vi "tap_stim_rec_async.vi"(0 "Convert Power to Voltage B":bool, 2 "voltages/power B":dbl[](array[numeric]), 3 "SSH password":string, 4 "Transfer and Run Date Folder After Experiment":bool, 5 "SSH user name":string, 6 "Tags":string, 7 "Frames":i32, 8 "Convert Power to Voltage":bool, 9 "voltages/power A":dbl[](array[numeric]), 10 "parameters":string[](array[string]), 11 "parameters headers":string[](array[string])) -> ()   [LabVIEW 2014]
uses:
  <vilib>/vision/driver/IMAQdx.llb/IMAQdx Acquisition Mode.ctl
  <vilib>/userdefined/High Color/IMAQdx.ctl
  <vilib>/vision/driver/IMAQdx.llb/IMAQdx Buffer Number Mode.ctl
  <vilib>/Utility/file.llb/Write To Spreadsheet File (DBL).vi
  <vilib>/Utility/file.llb/Write To Spreadsheet File (string).vi
  <vilib>/Utility/file.llb/Read From Spreadsheet File (string).vi
  <vilib>/vision/driver/NI_Vision_Acquisition_Software.lvlib
panel:
  out "Waveform Graph":dbl[](graph)
  out "Current Voltage B":dbl
  out "Current Voltage A":dbl
  out "Saved Buffer Number":u32
  out "ProcessFrameRate":dbl
  out "# elements in queue":i32
  out "CameraFrameRate":dbl
  out "Camera Buffer Number":u32
  out "Image":T1(plugin-control)
  out "JPEG Quality":dbl
  out "Error":string
  out "Save Directory":path
  in  "stop":bool
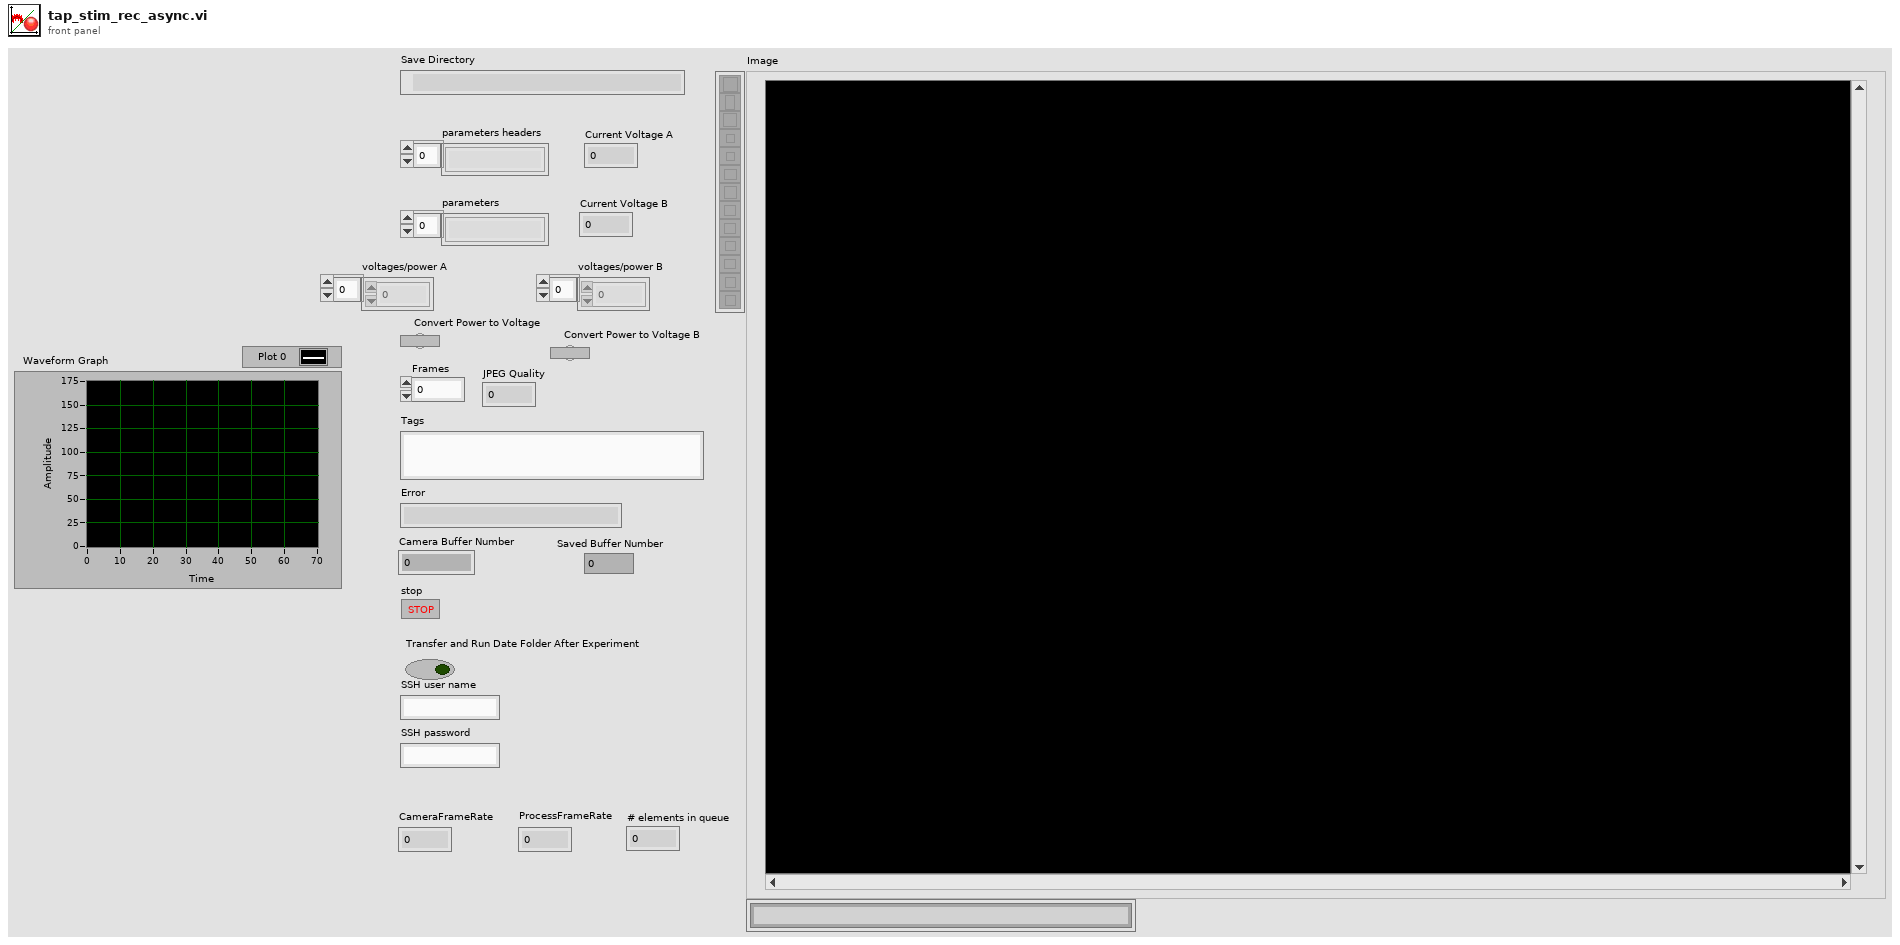
[diagram p1: front panel]
types:
  T1 = typedef "IMAQ Image.ctl" = refnum<image>
  T2 = typedef "IMAQdx.ctl" = refnum<k21>
  T3 = typedef "NI_Vision_Acquisition_Software.lvlib/IMAQdx Buffer Number Mode.ctl" = enum32{"Next", "Last", "Buffer Number"}
  T4 = typedef "Image Type" = u32
  T5 = typedef "NI_Vision_Acquisition_Software.lvlib/IMAQdx Acquisition Mode.ctl" = enum32{"One Shot", "Continuous"}
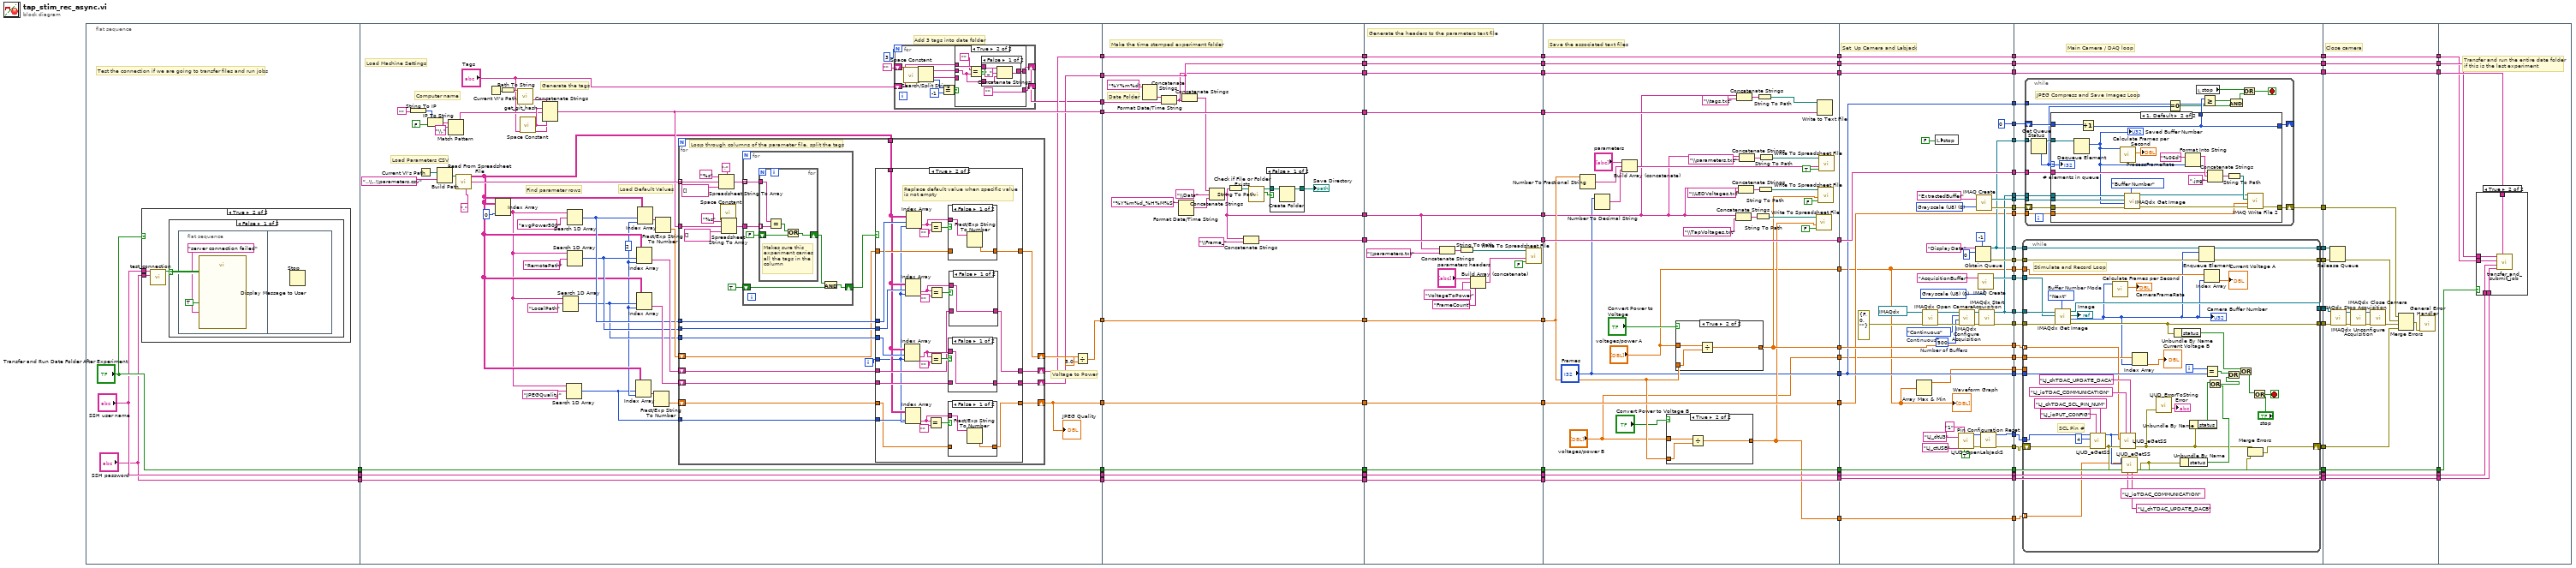
[diagram p0: block diagram]
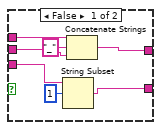
[diagram p4: hidden frame]
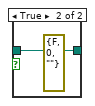
[diagram p11: hidden frame]
diagram:
  n1 = flat-sequence {
    tunnel: ["Transfer and Run Date Folder After Experiment"] -> w55
    tunnel: ["SSH user name"] -> w54
    tunnel: ["SSH password"] -> w53
    tunnel: [w139] -> w85
    tunnel: [w122] -> w84
    tunnel: [w113] -> w75
    tunnel: [w114] -> w74
    tunnel: w55 -> [w131]
    tunnel: w54 -> [w130]
    tunnel: w53 -> [w129]
    tunnel: [w131] -> w46
    tunnel: [w130] -> w39
    tunnel: [w129] -> w38
    tunnel: [w110] -> w31
    tunnel: [w101] -> w30
    tunnel: [w275] -> w69
    tunnel: [w274] -> w67
    tunnel: [w273] -> w65
    tunnel: [w272] -> w63
    tunnel: [w254] -> w61
    tunnel: [w256] -> w59
    tunnel: [w271] -> w57
    tunnel: w74 -> [w271]
    tunnel: w75 -> [w256]
    tunnel: w84 -> [w272]
    tunnel: w85 -> [w273]
    tunnel: [w263] -> w47
    tunnel: w46 -> [w263]
    tunnel: [w262] -> w40
    tunnel: w39 -> [w262]
    tunnel: w38 -> [w261]
    tunnel: [w261] -> w37
    tunnel: w31 -> [w257]
    tunnel: w30 -> [w253]
    tunnel: [w253] -> w27
    tunnel: w69 -> [w297]
    tunnel: [w297] -> w68
    tunnel: w67 -> [w283]
    tunnel: [w283] -> w66
    tunnel: w65 -> [w296]
    tunnel: [w296] -> w64
    tunnel: w63 -> [w295]
    tunnel: [w295] -> w62
    tunnel: w61 -> [w294]
    tunnel: [w294] -> w60
    tunnel: w59 -> [w293]
    tunnel: [w293] -> w58
    tunnel: w57 -> [w292]
    tunnel: [w292] -> w56
    tunnel: [w282] -> w48
    tunnel: w47 -> [w282]
    tunnel: [w281] -> w41
    tunnel: w40 -> [w281]
    tunnel: w37 -> [w280]
    tunnel: [w280] -> w36
    tunnel: [w279] -> w28
    tunnel: w27 -> [w279]
    tunnel: w68 -> [w332]
    tunnel: [w332] -> w90
    tunnel: [w302] -> w88
    tunnel: ["Frames"] -> w87
    tunnel: w66 -> [w303]
    tunnel: w64 -> [w309]
    tunnel: w62 -> [w312]
    tunnel: w60 -> [w321]
    tunnel: [w321] -> w80
    tunnel: [w320] -> w76
    tunnel: w58 -> [w320]
    tunnel: [w319] -> w70
    tunnel: w56 -> [w319]
    tunnel: [w315] -> w49
    tunnel: w48 -> [w315]
    tunnel: [w314] -> w42
    tunnel: w41 -> [w314]
    tunnel: w36 -> [w313]
    tunnel: [w313] -> w35
    tunnel: [w311] -> w29
    tunnel: w28 -> [w311]
    tunnel: [w301] -> w6
    tunnel: ["voltages/power A"] -> w5
    tunnel: ["voltages/power B"] -> w3
    tunnel: w90 -> [w352]
    tunnel: [w382] -> w92
    tunnel: [w381] -> w91
    tunnel: [w385] -> w89
    tunnel: w88 -> [w385]
    tunnel: w87 -> [w351]
    tunnel: [w351] -> w86
    tunnel: [w379] -> w81
    tunnel: w80 -> [w379]
    tunnel: [w378] -> w77
    tunnel: w76 -> [w378]
    tunnel: [w377] -> w71
    tunnel: w70 -> [w377]
    tunnel: [w376] -> w50
    tunnel: w49 -> [w376]
    tunnel: [w375] -> w43
    tunnel: w42 -> [w375]
    tunnel: w35 -> [w374]
    tunnel: [w374] -> w34
    tunnel: w29 -> [w349]
    tunnel: [w358] -> w26
    tunnel: [w353] -> w25
    tunnel: [w357] -> w24
    tunnel: [w356] -> w23
    tunnel: [w350] -> w22
    tunnel: [w355] -> w19
    tunnel: [w354] -> w18
    tunnel: [w353] -> w17
    tunnel: [w352] -> w16
    tunnel: [w351] -> w15
    tunnel: [w350] -> w14
    tunnel: [w349] -> w13
    tunnel: [0] -> w9
    tunnel: [w346] -> w7
    tunnel: w6 -> [w346]
    tunnel: w5 -> [w344]
    tunnel: [w344] -> w4
    tunnel: w3 -> [w345]
    tunnel: [w345] -> w2
    tunnel: [w343] -> w1
    tunnel: w92 -> [w406]
    tunnel: w91 -> [w398]
    tunnel: w89 -> [w404]
    tunnel: w86 -> [w405]
    tunnel: [w421] -> w82
    tunnel: w81 -> [w421]
    tunnel: [w420] -> w78
    tunnel: w77 -> [w420]
    tunnel: [w419] -> w72
    tunnel: w71 -> [w419]
    tunnel: [w418] -> w51
    tunnel: w50 -> [w418]
    tunnel: [w417] -> w44
    tunnel: w43 -> [w417]
    tunnel: w34 -> [w416]
    tunnel: [w416] -> w33
    tunnel: w26 -> [w399]
    tunnel: w25 -> [w400]
    tunnel: w24 -> [w401]
    tunnel: w23 -> [w402]
    tunnel: w22 -> [w403]
    tunnel: [w394] -> w21
    tunnel: [w393] -> w20
    tunnel: w19 -> [w415]
    tunnel: w18 -> [w414]
    tunnel: w17 -> [w413]
    tunnel: w16 -> [w412]
    tunnel: w15 -> [w411]
    tunnel: w14 -> [w410]
    tunnel: w13 -> [w409]
    tunnel: [w392] -> w12
    tunnel: [w395] -> w11
    tunnel: [w408] -> w10
    tunnel: w9 -> [w407]
    tunnel: [w396] -> w8
    tunnel: w7 -> [w397]
    tunnel: w4 -> [w391]
    tunnel: w2 -> [w390]
    tunnel: w1 -> [w389]
    tunnel: [w524] -> w83
    tunnel: w82 -> [w524]
    tunnel: [w523] -> w79
    tunnel: w78 -> [w523]
    tunnel: [w522] -> w73
    tunnel: w72 -> [w522]
    tunnel: [w521] -> w52
    tunnel: w51 -> [w521]
    tunnel: [w520] -> w45
    tunnel: w44 -> [w520]
    tunnel: w33 -> [w519]
    tunnel: [w519] -> w32
    tunnel: w21 -> [w514]
    tunnel: w20 -> [w513]
    tunnel: w12 -> [w508]
    tunnel: w11 -> [w511]
    tunnel: w10 -> [w510]
    tunnel: w8 -> [w509]
    tunnel: w83 -> [w530]
    tunnel: w79 -> [w529]
    tunnel: w73 -> [w528]
    tunnel: w52 -> [w527]
    tunnel: w45 -> [w526]
    tunnel: w32 -> [w525]
    frame #0 {
      # "Test the connection if we are going to transfer files and run jobs"
      n2 = case shown="True" "Transfer and Run Date Folder After Experiment" {
        tunnel: "SSH password" -> [_ w98]
        tunnel: "SSH user name" -> [_ w96]
        frame False {
        }
        frame True {
          n3 = call "test_connection.vi"("Username"=w96, "Password"=w98) -> ("Connection Successful"=w97:bool)  [unwired: 7 in]
          n4 = case shown="False" w97 {
            frame False {
              n5 = flat-sequence {
                frame #0 {
                  n6 = call "Display Message to User"("Enable"=TRUE, "Message"="server connection failed") -> ()  [unwired: 8 in, 2 out]
                }
                frame #1 {
                  n7 = Stop() -> ()  [unwired: 1 in]
                }
              }
            }
            frame True {
            }
          }
        }
      }
    }
    frame #1 {
      w104 = 2
      # "Add 3 tags into date folder"
      # "Generate the tags"
      # "Find parameter rows"
      # "Load Default Values"
      # "Voltage to Power"
      # "Load Parameters CSV"
      # "Computer name"
      # "Load Machine Settings"
      n8 = String To IP(1:"") -> (0:w147:u32)
      n9 = Current VI's Path() -> (path=w142:path)
      n10 = IP To String(1:FALSE, 2:w147) -> (0:w144:string)
      n11 = Build Path(base path=w142, name or relative path="..\\..\\parameters.csv") -> (appended path=w133:path)
      n12 = Match Pattern(string=w144, regular expression="\\.") -> (before substring=w124:string)  [unwired: 1 in, 3 out]
      n13 = call-poly <vilib>:"Read From Spreadsheet File.vi"("delimiter (\\t)"=",", "file path (dialog if empty)"=w133) -> ("first row"=w123:string[], "all rows"=w106:string[][])  [unwired: 5 in, 3 out]
      n14 = Current VI's Path() -> (path=w126:path)
      n15 = Index Array(array=w106, index (col)=0) -> (element=w105:string[])  [unwired: 1 in]
      n16 = Path To String(path=w126) -> (string=w125:string)
      n17 = call "get_git_hash.vi"("VI folder"=w125) -> ("github hash"=w128:string)  [unwired: 10 in]
      n18 = call <vilib>:"Space Constant.vi"() -> ("String"=w127:string)
      n19 = Concatenate Strings(w128, w127, w124, w127, "Tags") -> (w122:string)
      n20 = Search 1D Array(1D array=w105, element="LocalPath") -> (index of element=w116:i32)  [unwired: 1 in]
      n21 = Search 1D Array(1D array=w105, element="JPEGQuality") -> (index of element=w102:i32)  [unwired: 1 in]
      n22 = Search 1D Array(1D array=w105, element="RemotePath") -> (index of element=w117:i32)  [unwired: 1 in]
      n23 = Search 1D Array(1D array=w105, element="avgPower500") -> (index of element=w118:i32)  [unwired: 1 in]
      n24 = Index Array(array=w106, index (row)=w102, index (col)=w104) -> (element=w107:string)
      n25 = Index Array(array=w106, index (row)=w117, index (col)=w104) -> (element=w120:string)
      n26 = Index Array(array=w106, index (row)=w116, index (col)=w104) -> (element=w119:string)
      n27 = Index Array(array=w106, index (row)=w118, index (col)=w104) -> (element=w135:string)
      n28 = Fract/Exp String To Number(string=w107) -> (number=w103:dbl)  [unwired: 3 in, 1 out]
      n29 = Fract/Exp String To Number(string=w135) -> (number=w121:dbl)  [unwired: 3 in, 1 out]
      n30 = for {
        tunnel: w123 -> [w201] mode=indexing
        tunnel: w122 -> [w193]
        tunnel: w118 -> [w188]
        tunnel: w117 -> [w187]
        tunnel: w116 -> [w186]
        tunnel: w106 -> [w191]
        shift-right: [w183] -> w115
        shift-left: w121 -> [w184]
        shift-right: [w180] -> w114
        shift-left: w120 -> [w181]
        shift-right: [w179] -> w113
        shift-left: w119 -> [w182]
        shift-right: [w176] -> w101
        shift-left: w103 -> [w178]
        tunnel: w102 -> [w177]
        i -> [w185]
        # "Loop through columns of the parameter file, split the tags"
        n31 = Spreadsheet String To Array(delimiter (Tab)=";", format string="%s", spreadsheet string=w201, array type (2D Dbl)=string[] []) -> (array=w197:string[])
        n32 = call <vilib>:"Space Constant.vi"() -> ("String"=w195:string)
        n33 = Spreadsheet String To Array(delimiter (Tab)=w195, format string="%s", spreadsheet string=w193, array type (2D Dbl)=string[] []) -> (array=w192:string[])
        n34 = for {
          tunnel: w197 -> [w247] mode=indexing
          tunnel: w192 -> [w246]
          shift-right: [w244] -> w189
          shift-left: TRUE -> [w242]
          n35 = for {
            tunnel: w247 -> [w252]
            tunnel: w246 -> [w251] mode=indexing
            shift-right: [w248] -> w243
            shift-left: FALSE -> [w249]
            # "Makes sure this\nexperiment carries\nall the tags in the\ncolumn"
            n36 = Equal?(x=w252, y=w251) -> (x = y?=w250:bool)
            n37 = Or(x=w250, y=w249) -> (x .or. y?=w248:bool)
          }
          n38 = And(x=w243, y=w242) -> (x .and. y?=w244:bool)
        }
        n39 = case shown="True" w189 {
          tunnel: w184 -> [w205 w226]
          tunnel: [w205 w225] -> w183
          tunnel: w188 -> [_ w231]
          tunnel: w187 -> [_ w230]
          tunnel: w186 -> [_ w229]
          tunnel: w185 -> [_ w208]
          tunnel: w191 -> [_ w209]
          tunnel: [w204 w215] -> w180
          tunnel: [w203 w217] -> w179
          tunnel: w182 -> [w203 w216]
          tunnel: w181 -> [w204 w214]
          tunnel: w178 -> [w202 w206]
          tunnel: w177 -> [_ w207]
          tunnel: [w202 w210] -> w176
          frame False {
          }
          frame True {
            # "Replace default value when specific value\nis not empty"
            n40 = Index Array(array=w209, index (row)=w229, index (col)=w208) -> (element=w218:string)
            n41 = Index Array(array=w209, index (row)=w230, index (col)=w208) -> (element=w221:string)
            n42 = Index Array(array=w209, index (row)=w207, index (col)=w208) -> (element=w211:string)
            n43 = Index Array(array=w209, index (row)=w231, index (col)=w208) -> (element=w224:string)
            n44 = Equal?(x=w211, y="") -> (x = y?=w212:bool)
            n45 = Equal?(x=w224, y="") -> (x = y?=w227:bool)
            n46 = Equal?(x=w218, y="") -> (x = y?=w219:bool)
            n47 = Equal?(x=w221, y="") -> (x = y?=w222:bool)
            n48 = case shown="False" w212 {
              tunnel: w206 -> [_ w234]
              tunnel: [w233 w234] -> w210
              tunnel: w211 -> [w232 _]
              frame False {
                n49 = Fract/Exp String To Number(string=w232) -> (number=w233:dbl)  [unwired: 3 in, 1 out]
              }
              frame True {
              }
            }
            n50 = case shown="False" w227 {
              tunnel: w226 -> [_ w241]
              tunnel: [w240 w241] -> w225
              tunnel: w224 -> [w239 _]
              frame False {
                n51 = Fract/Exp String To Number(string=w239) -> (number=w240:dbl)  [unwired: 3 in, 1 out]
              }
              frame True {
              }
            }
            n52 = case shown="False" w219 {
              tunnel: w218 -> [w235 _]
              tunnel: [w235 w236] -> w217
              tunnel: w216 -> [_ w236]
              frame False {
              }
              frame True {
              }
            }
            n53 = case shown="False" w222 {
              tunnel: w221 -> [w237 _]
              tunnel: [w237 w238] -> w215
              tunnel: w214 -> [_ w238]
              frame False {
              }
              frame True {
              }
            }
          }
        }
      }
      "JPEG Quality" <- w101
      n54 = for {
        N: 3 -> [_]
        shift-right: [w148] -> _
        shift-left: "Tags" -> [w157]
        shift-right: [w150] -> w110
        shift-left: "" -> [w155]
        n55 = call <vilib>:"Space Constant.vi"() -> ("String"=w156:string)
        n56 = Search/Split String(string=w157, search string/char (-)=w156) -> (substring before match=w154:string, match + rest of string=w153:string, offset of match=w152:i32)  [unwired: 1 in]
        n57 = Equal?(x=w152, y=-1) -> (x = y?=w149:bool)
        n58 = case shown="True" w149 {
          tunnel: w155 -> [w158 w168]
          tunnel: w154 -> [w159 w165]
          tunnel: w153 -> [w160 _]
          tunnel: [w162 ""] -> w148
          tunnel: [w161 w167] -> w150
          frame False {
            n59 = String Subset(string=w160, offset (0)=1) -> (substring=w162:string)  [unwired: 1 in]
            n60 = Concatenate Strings(w158, "_", w159) -> (w161:string)
          }
          frame True {
            n61 = Equal?(x="", y=w165) -> (x = y?=w169:bool)
            n62 = case shown="False" w169 {
              tunnel: w168 -> [w172 w175]
              tunnel: [w173 w175] -> w167
              tunnel: w165 -> [w171 _]
              frame False {
                n63 = Concatenate Strings(w172, "_", w171) -> (w173:string)
              }
              frame True {
              }
            }
          }
        }
      }
      n64 = Divide(x=w115, y=5.0) -> (x/y=w139:dbl)
    }
    frame #2 {
      # "Make the time stamped experiment folder"
      # "Date Folder"
      n65 = Format Date/Time String(time format string (%c)="%Y%m%d") -> (date/time string=w258:string)  [unwired: 2 in]
      n66 = Concatenate Strings(w258, w257) -> (w254:string)
      n67 = Format Date/Time String(time format string (%c)="%Y%m%d_%H%M%S") -> (date/time string=w260:string)  [unwired: 2 in]
      n68 = Concatenate Strings(w256, w254) -> (w255:string)
      n69 = Concatenate Strings(w255, "\\Data", w260) -> (w274:string)
      n70 = String To Path(string=w274) -> (path=w266:path)
      n71 = Concatenate Strings(w274, "\\Frame_") -> (w275:string)
      n72 = call <vilib>:"Check if File or Folder Exists.vi"("path"=w266) -> ("file or folder exists?"=w269:bool, "dup path"=w268:path)  [unwired: 8 in, 1 out]
      n73 = case shown="False" w269 {
        tunnel: [w276 w278] -> w265
        tunnel: w268 -> [w277 w278]
        frame False {
          n74 = Create Folder(path (use dialog)=w277) -> (created path=w276:path)  [unwired: 2 in, 2 out]
        }
        frame True {
          (unwired) errorcluster {"status"=FALSE, "code"=0, "source"=""} ("error out")
        }
      }
      "Save Directory" <- w265
    }
    frame #3 {
      # "Generate the headers to the parameters text file"
      n75 = Concatenate Strings(w283, "\\parameters.txt") -> (w291:string)
      n76 = String To Path(string=w291) -> (path=w290:path)
      n77 = Build Array (concatenate)("parameters headers", "VoltageToPower", "FrameCount") -> (w287:string[])
      n78 = call-poly <vilib>:"Write To Spreadsheet File.vi"("append to file? (new file:F)"=FALSE, "1D data"=w287, "file path (dialog if empty)"=w290) -> ()  [unwired: 5 in, 1 out]
    }
    frame #4 {
      # "Save the associated text files"
      n79 = Number To Fractional String(number=w309) -> (F-format string=w316:string)  [unwired: 3 in]
      n80 = Number To Decimal String(number="Frames") -> (decimal integer string=w317:string)  [unwired: 1 in]
      n81 = Build Array (concatenate)("parameters", w316, w317) -> (w325:string[])
      n82 = case shown="True" "Convert Power to Voltage B" {
        tunnel: "voltages/power B" -> [w335 w338]
        tunnel: [w335 w336] -> w301
        tunnel: w309 -> [_ w337]
        frame False {
        }
        frame True {
          n83 = Divide(x=w338, y=w337) -> (x/y=w336:dbl[])
        }
      }
      n84 = case shown="True" "Convert Power to Voltage" {
        tunnel: "voltages/power A" -> [w339 w342]
        tunnel: [w339 w340] -> w302
        tunnel: w309 -> [_ w341]
        frame False {
        }
        frame True {
          n85 = Divide(x=w342, y=w341) -> (x/y=w340:dbl[])
        }
      }
      n86 = Concatenate Strings(w303, "\\TapVoltages.txt") -> (w307:string)
      n87 = Concatenate Strings(w303, "\\tags.txt") -> (w323:string)
      n88 = Concatenate Strings(w303, "\\LEDVoltages.txt") -> (w334:string)
      n89 = Concatenate Strings(w303, "\\parameters.txt") -> (w329:string)
      n90 = String To Path(string=w307) -> (path=w306:path)
      n91 = String To Path(string=w323) -> (path=w322:path)
      n92 = String To Path(string=w334) -> (path=w333:path)
      n93 = String To Path(string=w329) -> (path=w328:path)
      n94 = call-poly <vilib>:"Write To Spreadsheet File.vi"("append to file? (new file:F)"=FALSE, "1D data"=w301, "file path (dialog if empty)"=w306) -> ()  [unwired: 5 in, 1 out]
      n95 = Write to Text File(file (use dialog)=w322, text=w312) -> ()  [unwired: 2 in, 3 out]
      n96 = call-poly <vilib>:"Write To Spreadsheet File.vi"("append to file? (new file:F)"=FALSE, "1D data"=w302, "file path (dialog if empty)"=w333) -> ()  [unwired: 5 in, 1 out]
      n97 = call-poly <vilib>:"Write To Spreadsheet File.vi"("append to file? (new file:F)"=TRUE, "1D data"=w325, "file path (dialog if empty)"=w328) -> ()  [unwired: 5 in, 1 out]
    }
    frame #5 {
      w361 = T4 0 items=["Grayscale (U8)", "Grayscale (I16)", "Grayscale (SGL)", "Complex (CSG)", "RGB (U32)", "HSL (U32)", "RGB (U64)"] ("Image Type")
      w370 = T4 0 items=["Grayscale (U8)", "Grayscale (I16)", "Grayscale (SGL)", "Complex (CSG)", "RGB (U32)", "HSL (U32)", "RGB (U64)"] ("Image Type")
      w371 = u32 500  # Number of Buffers
      w367 = IMAQdx_Acquisition_Mode."Continuous"  # Continuous?
      # "Set  Up Camera and Labjack"
      n98 = Array Max & Min(array=w344) -> (max value=w343:dbl)  [unwired: 3 out]
      n99 = call <vilib>:"IMAQdx Open Camera.vi"("error in"=errorcluster {"status"=FALSE, "code"=0, "source"=""}, "Session In"=T2 "cam0") -> ("error out"=w372:errorcluster, "Session Out"=w373:T2)  [unwired: 8 in]
      n100 = local write "stop"(FALSE) -> ()
      n101 = call "LJUD_OpenLabJackS.vi"("FirstFound"=TRUE, "Address"="1" ("DeviceType"), "ConnectionType"="LJ_ctUSB", "DeviceType"="LJ_dtU3") -> ("error out"=w380:errorcluster, "Handle"=w383:i32)  [unwired: 5 in, 1 out]
      n102 = call <vilib>:"IMAQdx Configure Acquisition.vi"("error in"=w372, "Number of Buffers"=w371, "Continuous?"=w367, "Session In"=w373) -> ("error out"=w368:errorcluster, "Session Out"=w366:T2)  [unwired: 6 in]
      n103 = Obtain Queue(max queue size (-1, unlimited)=-1, name (unnamed)="DisplayData", element data type=u32 0) -> (queue out=w350:refnum<queue>, error out=w356:errorcluster)  [unwired: 2 in, 1 out]
      n104 = call "IMAQ Create"("Image Name"="ExtractedBuffer", "Image Type"=w361) -> ("New Image"=w354:T1, "error out"=w355:errorcluster)  [unwired: 3 in]
      n105 = call "IMAQ Create"("Image Name"="AcquisitionBuffer", "Image Type"=w370) -> ("New Image"=w357:T1)  [unwired: 3 in, 1 out]
      n106 = call <vilib>:"IMAQdx Start Acquisition.vi"("error in"=w368, "Session In"=w366) -> ("error out"=w358:errorcluster, "Session Out"=w353:T2)  [unwired: 8 in]
      n107 = call "Pin Configuration Reset.vi"("error in"=w380, "Handle In"=w383) -> ("error out"=w381:errorcluster, "Handle Out"=w382:i32)  [unwired: 8 in]
      "Waveform Graph" <- w344
    }
    frame #6 {
      # "Main Camera / DAQ loop"
      n108 = while {
        shift-right: [w427] -> w392
        shift-left: w398 -> [w455]
        tunnel: w404 -> [w454] mode=indexing
        tunnel: w405 -> [w461]
        tunnel: w399 -> [w450]
        tunnel: w400 -> [w449]
        tunnel: w401 -> [w448]
        tunnel: w402 -> [w447]
        tunnel: w403 -> [w446]
        tunnel: [w442] -> w396
        tunnel: [w441] -> w395
        tunnel: [w440] -> w394
        tunnel: [w439] -> w393
        tunnel: w406 -> [w435]
        tunnel: w397 -> [w433] mode=indexing
        tunnel: w391 -> [w425]
        tunnel: w390 -> [w423]
        tunnel: w389 -> [_]
        i -> [w462]
        stop <- w466 stop-if-true
        w453 = IMAQdx_Buffer_Number_Mode."Next"  # Buffer Number Mode
        # "Stimulate and Record Loop"
        # "SCL Pin #"
        n109 = call <vilib>:"IMAQdx Get Image.vi"("Buffer Number Mode (Next)"=w453, "error in"=w450, "Image In"=w448, "Session In"=w449) -> ("error out"=w439:errorcluster, "Buffer Number Out"=w422:u32, "Image Out"=→"Image":T1, "Session Out"=w440:T2)  [unwired: 4 in]
        "Camera Buffer Number" <- w422
        n110 = call "LJUD_eGetSS.vi"("Channel"="LJ_chTDAC_SCL_PIN_NUM", "IOType"="LJ_ioPUT_CONFIG", "error in"=w455, "Value Write"=4, "Handle In"=w435) -> ("error out"=w438:errorcluster, "Handle Out"=w434:i32)  [unwired: 4 in, 1 out]
        n111 = call <vilib>:"Calculate Frames per Second.vi"("Buffer Number"=w422) -> ("Processed Frames/s"=→"CameraFrameRate":dbl)  [unwired: 8 in, 2 out]
        n112 = call "LJUD_eGetSS.vi"("Channel"="LJ_chTDAC_UPDATE_DACA", "IOType"="LJ_ioTDAC_COMMUNICATION", "error in"=w438, "Value Write"=w454, "Handle In"=w434) -> ("error out"=w429:errorcluster)  [unwired: 4 in, 2 out]
        n113 = call "LJUD_eGetSS.vi"("Channel"="LJ_chTDAC_UPDATE_DACB", "IOType"="LJ_ioTDAC_COMMUNICATION", "error in"=w438, "Value Write"=w433, "Handle In"=w434) -> ("error out"=w428:errorcluster)  [unwired: 4 in, 2 out]
        n114 = Index Array(array=w423, index=w422) -> (element=→"Current Voltage B":dbl)
        n115 = call "LJUD_ErrorToString.vi"("error in"=w429) -> ("String"=→"Error":string)  [unwired: 10 in]
        n116 = Unbundle By Name(w439) -> ("status"=w445:bool)
        n117 = Unbundle By Name(w428) -> ("status"=w432:bool)
        n118 = Unbundle By Name(w429) -> ("status"=w431:bool)
        n119 = Enqueue Element(queue=w446, element=w422, error in (no error)=w447) -> (queue out=w442:refnum<queue>, error out=w441:errorcluster)  [unwired: 1 in, 1 out]
        n120 = Index Array(array=w425, index=w422) -> (element=→"Current Voltage A":dbl)
        n121 = Equal?(x=w462, y=w461) -> (x = y?=w463:bool)
        n122 = Or(x=w431, y=w432) -> (x .or. y?=w430:bool)
        n123 = Or(x=w463, y=w430) -> (x .or. y?=w444:bool)
        n124 = Or(x=w445, y=w444) -> (x .or. y?=w443:bool)
        n125 = Merge Errors(w429, w428) -> (w427:errorcluster)
        n126 = Or(x=w443, y="stop") -> (x .or. y?=w466:bool)
      }
      n127 = while {
        tunnel: w410 -> [w484]
        tunnel: w414 -> [w482]
        tunnel: w413 -> [w481]
        tunnel: w412 -> [w479]
        shift-right: [w478] -> w408
        shift-left: w415 -> [w480]
        tunnel: w411 -> [w471]
        tunnel: w409 -> [w476]
        shift-right: [w473] -> _
        shift-left: w407 -> [w474]
        stop <- w477 stop-if-true
        # "JPEG Compress and Save Images Loop"
        n128 = Get Queue Status(queue=w484) -> (queue out=w483:refnum<queue>, # elements in queue=w467:i32)  [unwired: 2 in, 6 out]
        n129 = case shown="1, Default" w467 {
          selector: w467 -> [_ w505]
          tunnel: w483 -> [_ w503]
          tunnel: w482 -> [_ w502]
          tunnel: w481 -> [_ w501]
          tunnel: w480 -> [w486 w500]
          tunnel: w479 -> [_ w494]
          tunnel: [w486 w490] -> w478
          tunnel: w476 -> [_ w489]
          tunnel: w474 -> [w485 w488]
          tunnel: [w485 w487] -> w473
          tunnel: [w485 w487] -> w472
          frame 0 {
          }
          frame 1, Default {
            n130 = Dequeue Element(queue=w503) -> (element=w491:u32)  [unwired: 2 in, 3 out]
            "Saved Buffer Number" <- w491
            n131 = Increment(x=w488) -> (x+1=w487:i32)
            n132 = call <vilib>:"Calculate Frames per Second.vi"("Buffer Number"=w491) -> ("Processed Frames/s"=→"ProcessFrameRate":dbl)  [unwired: 8 in, 2 out]
            n133 = call <vilib>:"IMAQdx Get Image.vi"("Buffer Number Mode (Next)"=IMAQdx_Buffer_Number_Mode."Buffer Number", "error in"=w500, "Buffer Number In"=w491, "Image In"=w502, "Session In"=w501) -> ("error out"=w492:errorcluster, "Image Out"=w493:T1)  [unwired: 3 in, 2 out]
            n134 = Format Into String(format string="%06d" ("string"), w491) -> (resulting string=w496:string)  [unwired: 2 in, 1 out]
            n135 = Concatenate Strings(w494, w496, ".jpg" ("string")) -> (w498:string)
            n136 = String To Path(string=w498) -> (path=w497:path)
            n137 = call-poly "IMAQ Write File 2"("error in (no error)"=w492, "Image Quality"=w489, "File Path"=w497, "Image"=w493) -> ("error out"=w490:errorcluster)  [unwired: 6 in, 1 out]
            "# elements in queue" <- w505
          }
        }
        n138 = Equal To 0?(x=w467) -> (x = 0?=w468:bool)
        n139 = local read "stop"() -> (w475:bool)
        n140 = Greater Or Equal?(x=w472, y=w471) -> (x >= y?=w470:bool)
        n141 = And(x=w470, y=w468) -> (x .and. y?=w469:bool)
        n142 = Or(x=w475, y=w469) -> (x .or. y?=w477:bool)
      }
    }
    frame #7 {
      # "Close camera"
      n143 = Release Queue(queue=w509) -> ()  [unwired: 2 in, 3 out]
      n144 = call <vilib>:"IMAQdx Stop Acquisition.vi"("error in"=w513, "Session In"=w514) -> ("error out"=w515:errorcluster, "Session Out"=w516:T2)  [unwired: 8 in]
      n145 = call <vilib>:"IMAQdx Unconfigure Acquisition.vi"("error in"=w515, "Session In"=w516) -> ("error out"=w518:errorcluster, "Session Out"=w517:T2)  [unwired: 8 in]
      n146 = call <vilib>:"IMAQdx Close Camera.vi"("error in"=w518, "Session In"=w517) -> ("error out"=w507:errorcluster)  [unwired: 9 in]
      n147 = Merge Errors(w510, w511, w507, w508) -> (w512:errorcluster)
      n148 = call <vilib>:"General Error Handler.vi"("error in (no error)"=w512) -> ()  [unwired: 10 in, 5 out]
    }
    frame #8 {
      # "Transfer and run the entire date folder\nif this is the last experiment"
      n149 = case shown="True" w527 {
        tunnel: w530 -> [_ w535]
        tunnel: w529 -> [_ w534]
        tunnel: w528 -> [_ w533]
        tunnel: w526 -> [_ w532]
        tunnel: w525 -> [_ w531]
        frame False {
        }
        frame True {
          n150 = call "transfer_and_submit_job.vi"("Date Folder"=w535, "Password"=w531, "Username"=w532, "Remote Data Directory"=w533, "Local Data Directory"=w534) -> ()  [unwired: 7 in]
        }
      }
    }
  }
